vi "Enable Control.vi"(8 "error in (no error)":errorcluster, 11 "Ctrl Reference's in":refnum<class "Ctrl Reference's.lvclass">) -> (0 "error out":errorcluster, 3 "Ctrl Reference's out":refnum<class "Ctrl Reference's.lvclass">)   [LabVIEW 2020, in "Ctrl Reference's.lvclass"]
uses:
  Ctrl Reference's.lvclass
  Ctrl Reference's.lvclass/Ctrl Reference's.ctl
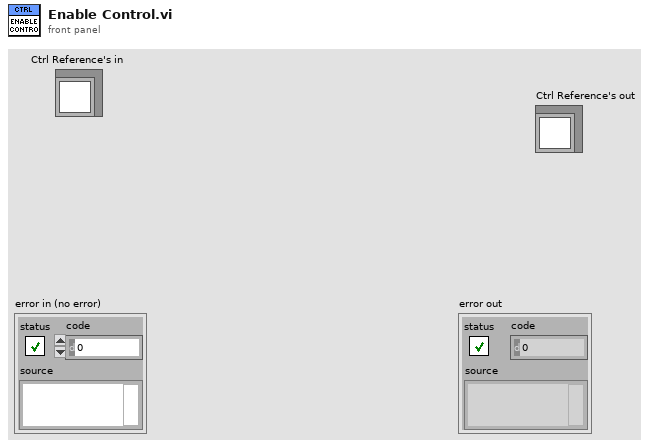
[diagram p1: front panel]
types:
  T1 = enum8{"Enabled", "Disabled", "Disabled and Grayed Out"}
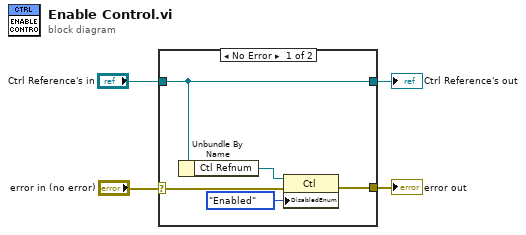
[diagram p0: block diagram]
diagram:
  n1 = case shown="No Error" "error in (no error)" {
    selector: "error in (no error)" -> [w6 w10]
    tunnel: [w9 w11] -> w3
    tunnel: "Ctrl Reference's in" -> [w9 w11]
    tunnel: [w5 w10] -> w1
    frame No Error {
      n2 = Unbundle By Name(w9) -> ("Ctl Refnum"=w8:refnum<vi>)
      n3 = property class="Ctl"(reference=w8, error in=w6, "DisabledEnum"=T1."Enabled" ("Disabled")) -> (error out=w5:errorcluster)  [unwired: 1 out]
    }
    frame Error {
    }
  }
  "Ctrl Reference's out" <- w3
  "error out" <- w1
